vi "Single Match Cluster to CSV Array.vi"(11 "Match Cluster":T1) -> (3 "csv array":string[][](array[string]))   [LabVIEW 2015]
uses:
  Typedef/JSONCluster.ctl
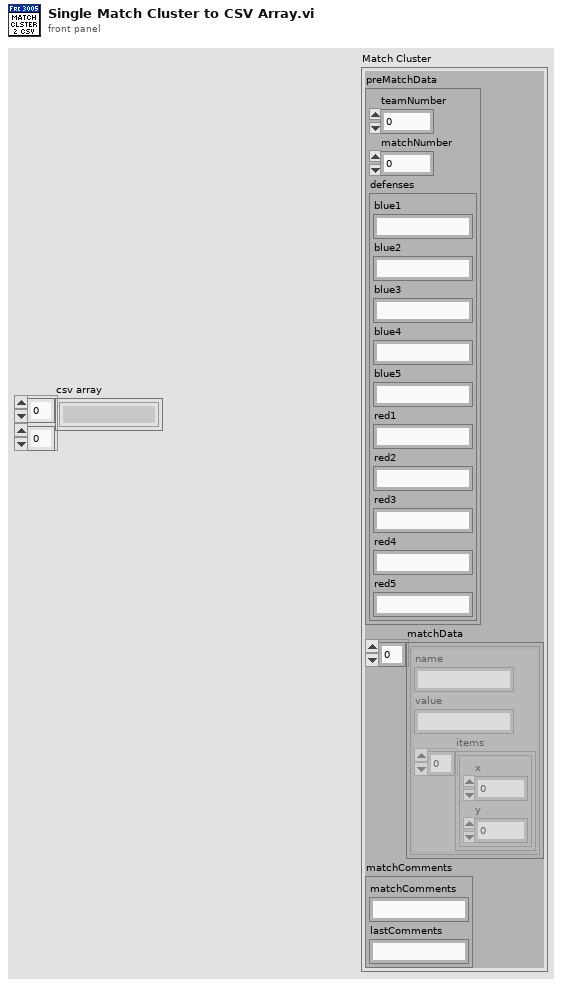
[diagram p1: front panel]
types:
  T1 = typedef "JSONCluster.ctl" = cluster{"preMatchData":cluster{"teamNumber":i32, "matchNumber":i32, "defenses":cluster{"blue1":string, "blue2":string, "blue3":string, "blue4":string, "blue5":string, "red1":string, "red2":string, "red3":string, "red4":string, "red5":string}}, "matchData":cluster{"name":string, "value":string, "items":cluster{"x":i32, "y":i32}[]}[], "matchComments":cluster{"matchComments":string, "lastComments":string}}
  T2 = cluster{"name":string, "value":string, "items":cluster{"x":i32, "y":i32}[]}[]
  T3 = cluster{"teamNumber":i32, "matchNumber":i32, "defenses":cluster{"blue1":string, "blue2":string, "blue3":string, "blue4":string, "blue5":string, "red1":string, "red2":string, "red3":string, "red4":string, "red5":string}}
  T4 = cluster{"blue1":string, "blue2":string, "blue3":string, "blue4":string, "blue5":string, "red1":string, "red2":string, "red3":string, "red4":string, "red5":string}
  T5 = cluster{"name":string, "value":string, "items":cluster{"x":i32, "y":i32}[]}
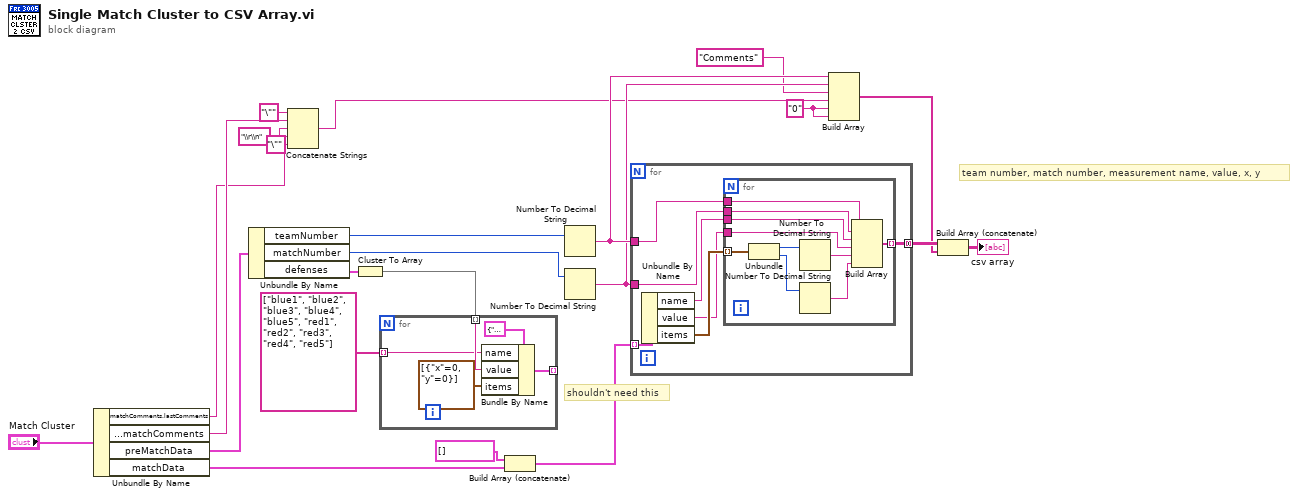
[diagram p0: block diagram]
diagram:
  w13 = "0" ("element")
  # "shouldn't need this"
  # "team number, match number, measurement name, value, x, y"
  n1 = Unbundle By Name("Match Cluster") -> ("matchComments.lastComments"=w15:string, "matchComments.matchComments"=w16:string, "preMatchData"=w23:T3, "matchData"=w6:T2)
  n2 = Unbundle By Name(w23) -> ("teamNumber"=w22:i32, "matchNumber"=w21:i32, "defenses"=w4:T4)
  n3 = Concatenate Strings("\"" ("string"), w16, "\\r\\n" ("string"), w15, "\"" ("string")) -> (w14:string)
  n4 = Cluster To Array(cluster=w4) -> (array=w3:string[])
  n5 = for {
    tunnel: w3 -> [w26] mode=indexing
    tunnel: string[] ["blue1", "blue2", "blue3", "blue4", "blue5", "red1", "red2", "red3", "red4", "red5"] -> [w25] mode=indexing
    tunnel: [w24] -> _ mode=indexing
    n6 = Bundle By Name(cluster=T5 {"name"="", "value"="", "items"=[]}, "name"=w25, "value"=w26, "items"=cluster{"x":i32, "y":i32}[] [{"x"=0, "y"=0}]) -> (w24:T5)
  }
  n7 = Build Array (concatenate)(T2 [] ("array"), w6) -> (w5:T2)
  n8 = Number To Decimal String(number=w22) -> (decimal integer string=w20:string)  [unwired: 1 in]
  n9 = Number To Decimal String(number=w21) -> (decimal integer string=w19:string)  [unwired: 1 in]
  n10 = for {
    tunnel: w5 -> [w35] mode=indexing
    tunnel: w20 -> [w31]
    tunnel: w19 -> [w30]
    tunnel: [w29] -> w12 mode=concatenating
    n11 = Unbundle By Name(w35) -> ("name"=w33:string, "value"=w32:string, "items"=w34:cluster{"x":i32, "y":i32}[])
    n12 = for {
      tunnel: w34 -> [w45] mode=indexing
      tunnel: w33 -> [w39]
      tunnel: w32 -> [w40]
      tunnel: w31 -> [w38]
      tunnel: w30 -> [w37]
      tunnel: [w36] -> w29 mode=indexing
      n13 = Unbundle(w45) -> ("x"=w44:i32, "y"=w43:i32)
      n14 = Number To Decimal String(number=w44) -> (decimal integer string=w41:string)  [unwired: 1 in]
      n15 = Number To Decimal String(number=w43) -> (decimal integer string=w42:string)  [unwired: 1 in]
      n16 = Build Array(w38, w37, w39, w40, w41, w42) -> (w36:string[])
    }
  }
  n17 = Build Array(w20, w19, "Comments" ("element"), w14, w13, w13) -> (w11:string[])
  n18 = Build Array (concatenate)(w12, w11) -> (→"csv array":string[][])
